vi "ViewCtl.vi"(8 "error in":errorcluster caption="错误输入（无错误）", 9 "禁用":u32, 10 "T？":bool, 11 "BoolIn":refnum<vi>) -> (0 "error out":errorcluster caption="错误输出")   [LabVIEW 2013]
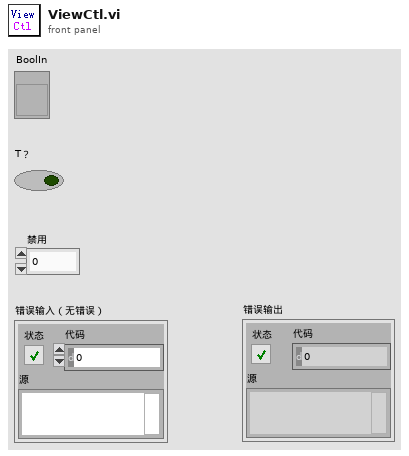
[diagram p1: front panel]
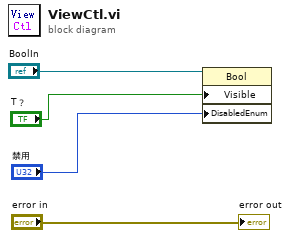
[diagram p0: block diagram]
diagram:
  n1 = property class="Bool"(reference="BoolIn", "Visible"="T？", "DisabledEnum"="禁用") -> ()  [unwired: 1 in, 2 out]
  "error out" <- "error in"
